vi "Core Read DAQ DVR FIFO.vi"(8 "error in (no error)":errorcluster, 9 "Timeout (ms)":i32=100, 10 "Data In":refnum<data-value>[](array[refnum]), 11 "CIFTag in":refnum<class "CIF_NIChn_Fifo_DAQ.lvclass">) -> (0 "error out":errorcluster, 1 "timed out?":bool, 2 "Data Out":refnum<data-value>[](array[refnum]), 3 "CIFTag out":refnum<class "CIF_NIChn_Fifo_DAQ.lvclass">, 4 "Header":T1)   [LabVIEW 2021, in "CIF_NIChn_Fifo_DAQ.lvclass"]
uses:
  CIF_NIChn_Fifo_DAQ.lvclass
  CIFChannels/Typedef/Direction.ctl
  CIFChannels/CIFChannels.lvclass
  CIFChannels/Typedef/Channel State.ctl
  NIChn/CIF_NIChn.lvclass
  <vilib>/CIF Foundation/CIF Channels/CIFChannels/CIFChannelCore.lvlib
  D:/dev/Packages/Channel_Manager/src/CIF_NIChn/NIChn/CIF_NIChn.lvclass
  D:/dev/Packages/Channel_Manager/src/CIFChannels/CIFChannels.lvclass
  ChannelCommon/ChannelCommon.lvlib
  683dda70-af16-44bc-a524-9971cb6dbe1c.vi
  9ab161bc-d75a-4f10-a981-8d657be3a6b1.vi
  ChannelCommon/typedef/FIFO Header.ctl
  ChannelCommon/typedef/Datatype Waveform.ctl
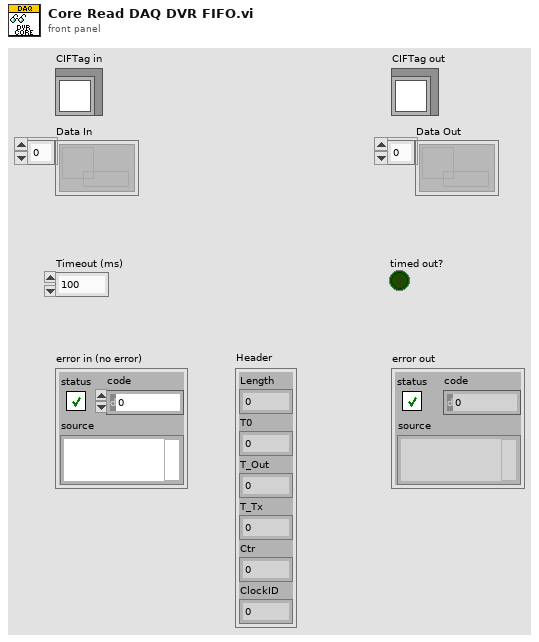
[diagram p1: front panel]
types:
  T1 = typedef "ChannelCommon.lvlib/FIFO Header.ctl" = cluster{"Length":u64, "T0":i64, "T_Out":i64, "T_Tx":i64, "Ctr":u64, "ClockID":u8}
  T2 = typedef "CIFChannels.lvclass/Channel State.ctl" = enum16{"Creating", "Disconnected", "Connecting", "Connected", "Destroyed"}
  T3 = typedef "CIFChannels.lvclass/Direction.ctl" = enum16{"Publisher", "Subscriber"}
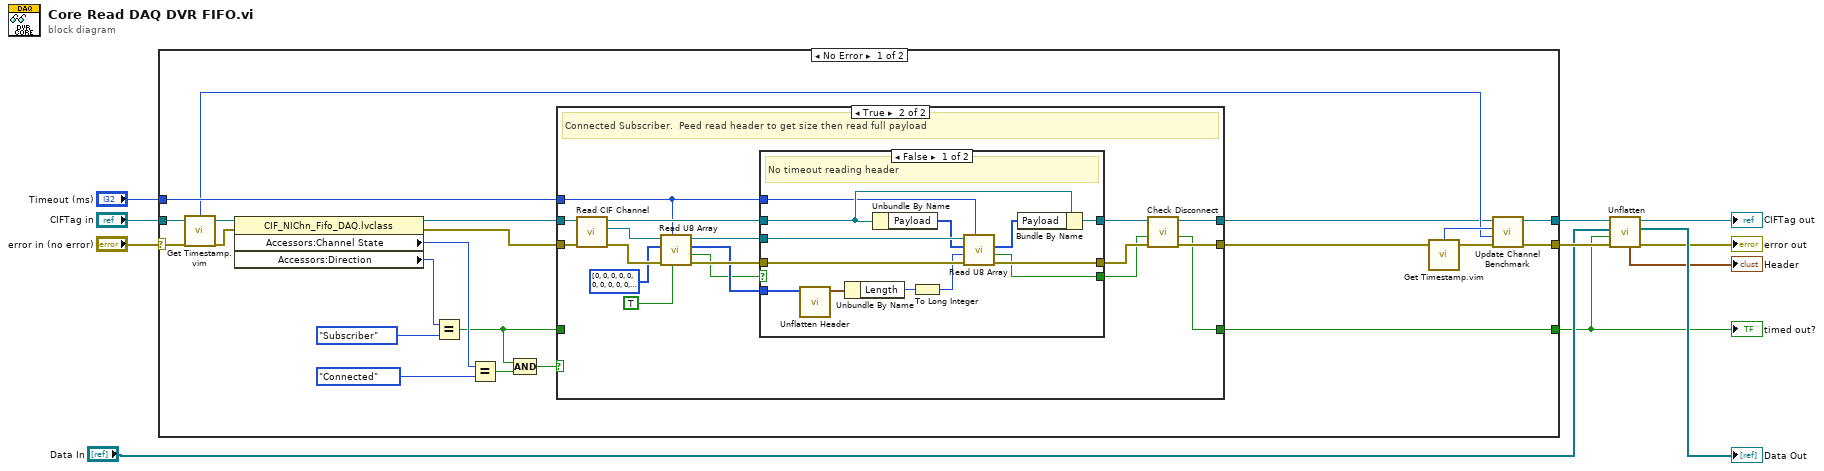
[diagram p0: block diagram]
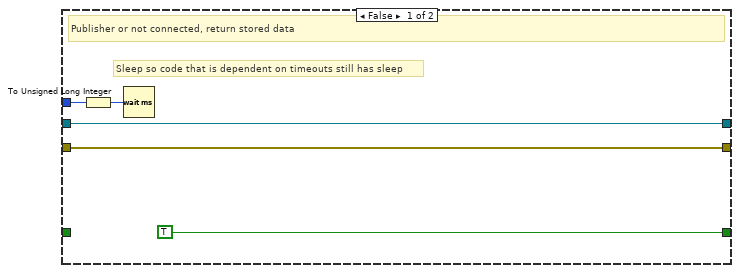
[diagram p2: hidden frame]
diagram:
  n1 = case shown="No Error" "error in (no error)" {
    selector: "error in (no error)" -> [w19 w73]
    tunnel: [w20 w73] -> w7
    tunnel: [w21 w72] -> w8
    tunnel: "CIFTag in" -> [w18 w72]
    tunnel: [w32 _] -> w1
    tunnel: "Timeout (ms)" -> [w22 _]
    frame No Error {
      n2 = call "Get Timestamp.vim"("Anything in"=w18) -> ("Time (ns)"=w15:i64, "Anything out"=w17:refnum<class "CIF_NIChn_Fifo_DAQ.lvclass">)  [unwired: 2 in]
      n3 = property class="CIF_NIChn_Fifo_DAQ.lvclass"(reference=w17, error in=w19) -> (reference out=w31:refnum<class "CIF_NIChn_Fifo_DAQ.lvclass">, error out=w30:errorcluster, "Accessors:Channel State"=w27:T2, "Accessors:Direction"=w29:T3)
      n4 = Equal?(x=w29, y=Direction."Subscriber") -> (x = y?=w23:bool)
      n5 = Equal?(x=w27, y=Channel_State."Connected") -> (x = y?=w25:bool)
      n6 = Compound Arithmetic op=AND(w23, w25) -> (w24:bool)
      n7 = case shown="True" w24 {
        tunnel: [TRUE ("timeout out") w48] -> w32
        tunnel: w30 -> [w36 w54]
        tunnel: w31 -> [w37 w55]
        tunnel: w23 -> [_ _]
        tunnel: [w37 w53] -> w13
        tunnel: [w36 w52] -> w12
        tunnel: w22 -> [w34 w38]
        frame False {
          # "Sleep so code that is dependent on timeouts still has sleep"
          # "Publisher or not connected, return stored data"
          n8 = To Unsigned Long Integer(number=w34) -> (unsigned 32bit integer=w33:u32)
          n9 = Wait (ms)(milliseconds to wait=w33) -> ()  [unwired: 1 out]
        }
        frame True {
          # "Connected Subscriber.  Peed read header to get size then read full payload"
          n10 = call "Read CIF Channel.vi"("error in (no error)"=w54, "CIFTag in"=w55) -> ("error out"=w49:errorcluster, "CIF Channel"=w50:refnum<k21>, "CIFTag out"=w51:refnum<class "CIF_NIChn_Fifo_DAQ.lvclass">)  [unwired: 7 in]
          n11 = call <vilib>:"Read U8 Array.vi"("Peek?"=TRUE, "Timeout (ms)"=w38, "error in"=w49, "U8 Array in"=u8[] [0, 0, 0, 0, 0, 0, 0, 0, 0, 0, 0, 0, 0, 0, 0, 0, 0, 0, 0, 0, 0, 0, 0, 0, 0, 0, 0, 0, 0, 0, 0, 0, 0, 0, 0, 0, 0, 0, 0, 0, 0, 0, 0, 0, 0, 0, 0, 0], "CIF Channel in"=w50) -> ("error out"=w46:errorcluster, "Timed out?"=w40:bool, "U8 Array out"=w43:u8[], "CIF Channel out"=w47:refnum<k21>)  [unwired: 3 in]
          n12 = case shown="False" w40 {
            selector: w40 -> [_ w71]
            tunnel: w51 -> [w68 w70]
            tunnel: w47 -> [w67 _]
            tunnel: w46 -> [w66 w69]
            tunnel: w43 -> [w63 _]
            tunnel: [w61 w69] -> w42
            tunnel: [w60 w70] -> w41
            tunnel: [w57 w71] -> w39
            tunnel: w38 -> [w56 _]
            frame False {
              # "No timeout reading header"
              n13 = call "Unflatten Header.vi"("Flattened Data in"=w63) -> ("Header out"=w62:T1)  [unwired: 8 in, 2 out]
              n14 = Unbundle By Name(w62) -> ("Length"=w59:u64)
              n15 = Unbundle By Name(w68) -> ("Payload"=w64:u8[])
              n16 = To Long Integer(number=w59) -> (32bit integer=w58:i32)
              n17 = call <vilib>:"Read U8 Array.vi"("Timeout (ms)"=w56, "error in"=w66, "Number of Elements"=w58, "U8 Array in"=w64, "CIF Channel in"=w67) -> ("error out"=w61:errorcluster, "Timed out?"=w57:bool, "U8 Array out"=w65:u8[])  [unwired: 3 in, 1 out]
              n18 = Bundle By Name(cluster=w68, "Payload"=w65) -> (w60:refnum<class "CIF_NIChn_Fifo_DAQ.lvclass">)
            }
            frame True {
              # "Timeout reading header"
            }
          }
          n19 = call "Check Disconnect.vi"("error in (no error)"=w42, "timeout in"=w39, "CIFTag in"=w41) -> ("error out"=w52:errorcluster, "timeout out"=w48:bool, "CIFTag out"=w53:refnum<class "CIF_NIChn_Fifo_DAQ.lvclass">)  [unwired: 5 in, 1 out]
        }
      }
      n20 = call "Get Timestamp.vim"("Anything in"=w12) -> ("Time (ns)"=w16:i64, "Anything out"=w14:errorcluster)  [unwired: 2 in]
      n21 = call "Update Channel Benchmark.vi"("error in (no error)"=w14, "X0"=w15, "X1"=w16, "CIFChannels in"=w13) -> ("error out"=w20:errorcluster, "CIFChannels out"=w21:refnum<class "CIF_NIChn_Fifo_DAQ.lvclass">)  [unwired: 6 in]
    }
    frame Error {
    }
  }
  "timed out?" <- w1
  n22 = call "Unflatten.vi"("error in (no error)"=w7, "timeout in"=w1, "Data In"="Data In", "CIFFifoCAN in"=w8) -> ("error out"=→"error out":errorcluster, "Data Out"=→"Data Out":refnum<data-value>[], "CIFFifoCAN out"=→"CIFTag out":refnum<class "CIF_NIChn_Fifo_DAQ.lvclass">, "Header"=→"Header":T1)  [unwired: 4 in]
